vi "Find Resource by Type (String).vi"(6 "Error if not found? (F)":bool, 8 "Error in":errorcluster caption="Error in (no error)", 10 "Resource Type":string, 11 "Resources":T2) -> (0 "Error out":errorcluster, 1 "Index":i32, 2 "Found?":bool, 3 "Resource":T1)   [LabVIEW 2018, in "Resource Manipulation.lvlib"]
uses:
  Resource Manipulation.lvlib
  Resource Array.ctl
  Resource.ctl
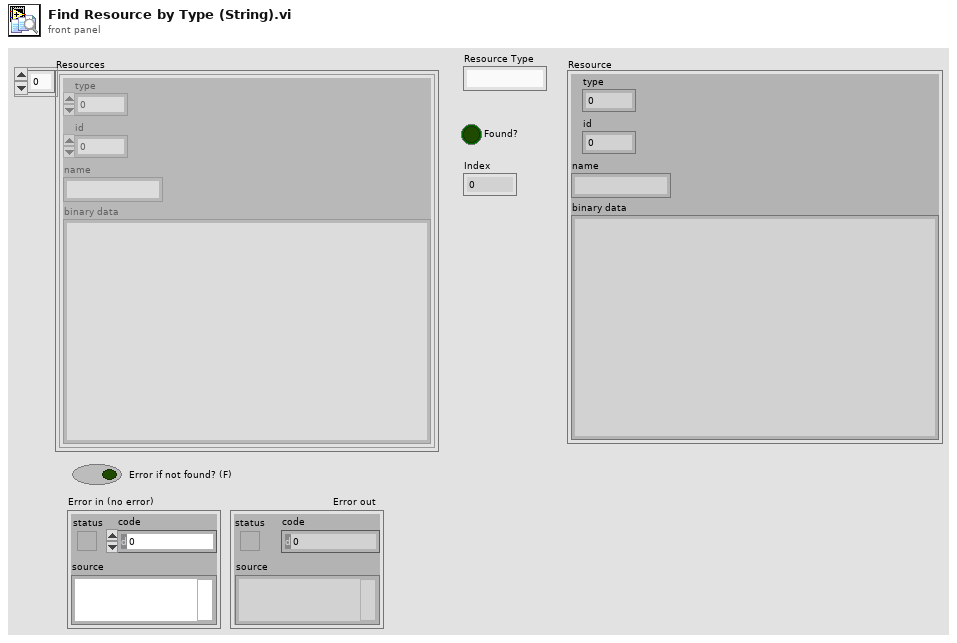
[diagram p1: front panel]
types:
  T1 = typedef "Resource Manipulation.lvlib/Resource.ctl" = cluster{"type":u32, "id":i32, "name":string, "binary data":string}
  T2 = typedef "Resource Manipulation.lvlib/Resource Array.ctl" = T1[]
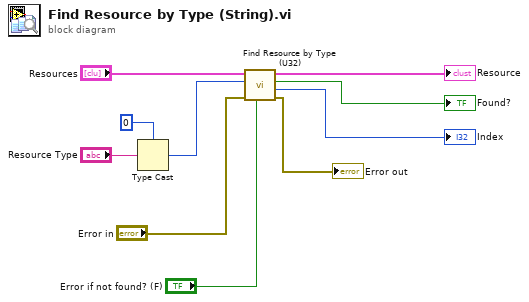
[diagram p0: block diagram]
diagram:
  n1 = Type Cast(type=u32 0 ("Resource Type"), x="Resource Type") -> (*(type *) &x=w7:u32)
  n2 = call "Find Resource by Type (U32).vi"("Error if not found? (F)"="Error if not found? (F)", "Error in"="Error in", "Resource Type"=w7, "Resources"="Resources") -> ("Error out"=→"Error out":errorcluster, "Index"=→"Index":i32, "Found?"=→"Found?":bool, "Resource"=→"Resource":T1)  [unwired: 4 in]
